vi "From Variant.vi"(0 "KObject in":refnum<class "KObject.lvclass">, 7 "Variant":variant, 9 "Prefix":string, 11 "error in (no error)":errorcluster) -> (4 "KObject out":refnum<class "KObject.lvclass">, 15 "error out":errorcluster)   [LabVIEW 2020, in "KObject.lvclass"]
uses:
  KObject.lvclass
  KObject.lvclass/KObject.ctl
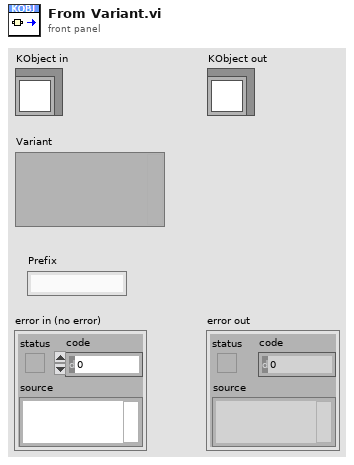
[diagram p1: front panel]
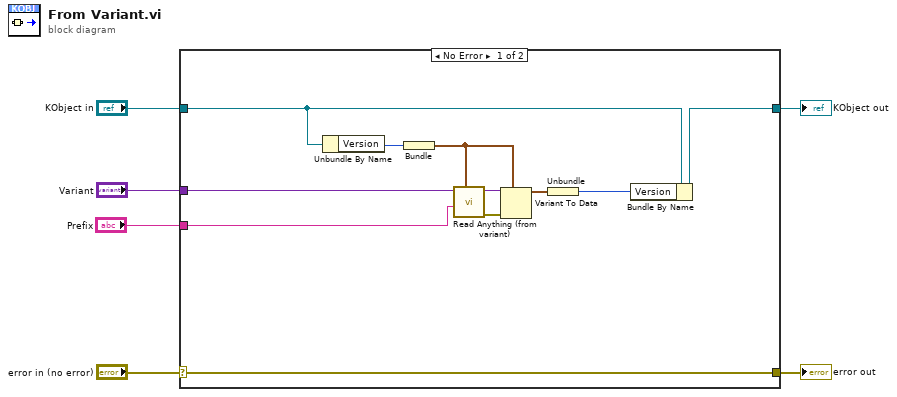
[diagram p0: block diagram]
diagram:
  n1 = case shown="No Error" "error in (no error)" {
    selector: "error in (no error)" -> [w17 w19]
    tunnel: [w17 w19] -> w5
    tunnel: [w9 w18] -> w3
    tunnel: "KObject in" -> [w16 w18]
    tunnel: "Variant" -> [w12 _]
    tunnel: "Prefix" -> [w7 _]
    frame No Error {
      n2 = Unbundle By Name(w16) -> ("Version"=w15:i32)
      n3 = Bundle("Version"=w15) -> (w11:cluster{"Version":i32})  [unwired: 1 in]
      n4 = call "Read Anything (from variant).vi"("Type of Anything"=w11, "Prefix"=w7, "Variant Database"=w12) -> ("Error Out"=w14:errorcluster, "Anything"=w13:variant)  [unwired: 6 in, 1 out]
      n5 = Variant To Data(error in=w14, type=w11, Variant=w13) -> (data=w10:cluster{"Version":i32})  [unwired: 1 out]
      n6 = Unbundle(w10) -> ("Version"=w8:i32)
      n7 = Bundle By Name(cluster=w16, "Version"=w8) -> (w9:refnum<class "KObject.lvclass">)
    }
    frame Error {
    }
  }
  "error out" <- w5
  "KObject out" <- w3
